vi "Authenticate user.vi"(8 "error in":errorcluster caption="에러 입력(에러 없음)", 9 "Password":string, 10 "User ID":string) -> (0 "error out":errorcluster caption="에러 출력", 1 "Verified?":bool)   [LabVIEW 2020]
uses:
  <vilib>/Utility/error.llb/DialogType.ctl
  <vilib>/addons/database/Connection.llb/Conn Execute.vi
  <vilib>/addons/database/Recordset.llb/Rec Get Recordset Properties (R).vi
  Variables/Global_Cal Info.vi
  <vilib>/addons/database/Recordset.llb/Rec Fetch String Data (R).vi
  <vilib>/addons/database/Recordset.llb/Rec Destroy - Connection.vi
  <vilib>/addons/database/NI_Database_API.lvlib
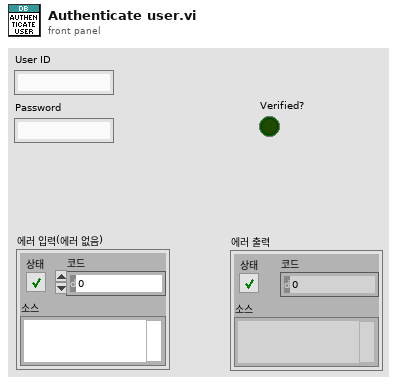
[diagram p1: front panel]
types:
  T1 = typedef "DialogType.ctl" = u16
  T2 = typedef "NI_Database_API.lvlib/Conn ObjectReference.ctl" = refnum<k1>
  T3 = typedef "NI_Database_API.lvlib/Rec ObjectReference.ctl" = refnum<k1>
  T4 = typedef "NI_Database_API.lvlib/Rec Properties.ctl" = cluster{"column count":i32, "record index":i32, "record count":i32, "bof?":bool, "eof?":bool, "cursor type":T5, "cache size":i32, "state":enum16{"closed", "open"}}
  T5 = typedef "NI_Database_API.lvlib/DB Tools Cursor Type.ctl" = enum16{"forward-only", "keyset", "dynamic", "static"}
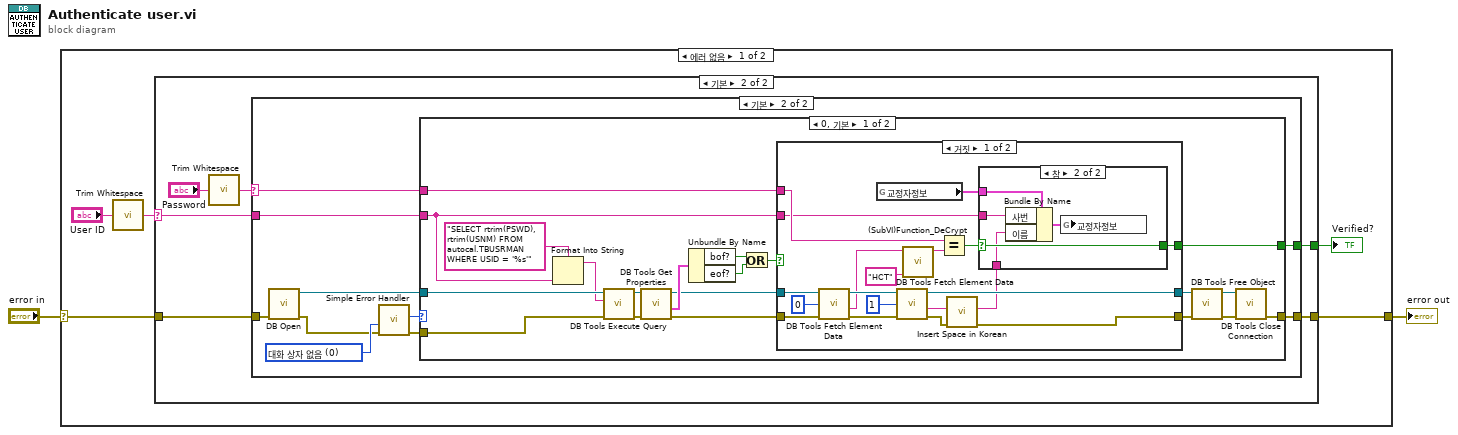
[diagram p0: block diagram]
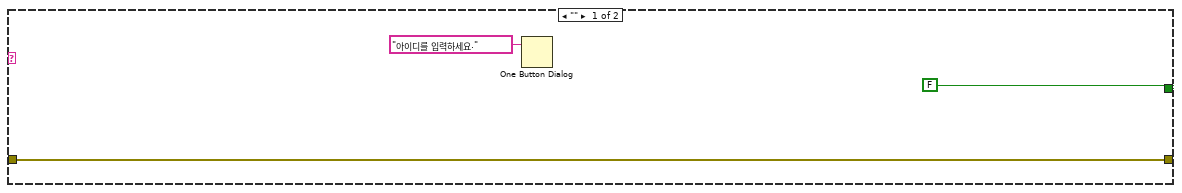
[diagram p2: hidden frame]
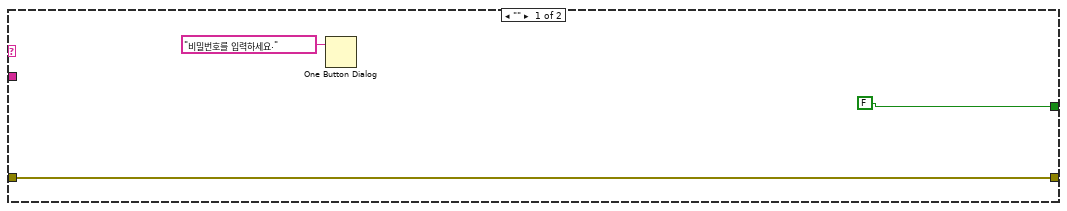
[diagram p3: hidden frame]
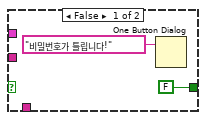
[diagram p4: hidden frame]
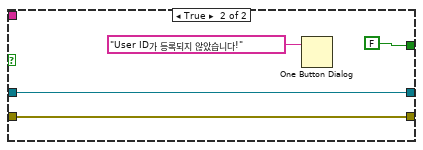
[diagram p5: hidden frame]
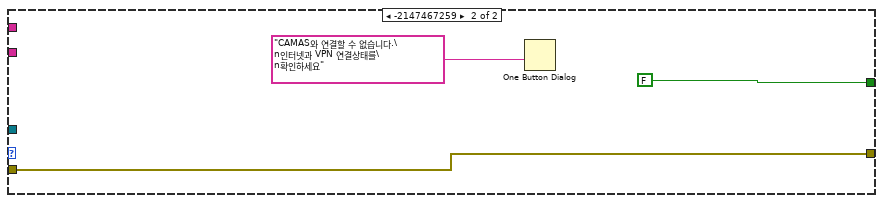
[diagram p6: hidden frame]
diagram:
  n1 = case shown="에러 없음" "error in" {
    selector: "error in" -> [w5 w83]
    tunnel: [w6 w83] -> w2
    frame No Error {
      n2 = call <vilib>:"Trim Whitespace.vi"("string"="User ID") -> ("trimmed string"=w3:string)  [unwired: 1 in]
      n3 = case shown="기본" w3 {
        selector: w3 -> [_ w13]
        tunnel: [w9 w16] -> w6
        tunnel: w5 -> [w9 w15]
        tunnel: [FALSE w14] -> w4
        frame "" {
          n4 = One Button Dialog(message="아이디를 입력하세요." ("메시지")) -> ()  [unwired: 1 in, 1 out]
        }
        frame Default {
          n5 = call <vilib>:"Trim Whitespace.vi"("string"="Password") -> ("trimmed string"=w11:string)  [unwired: 1 in]
          n6 = case shown="기본" w11 {
            selector: w11 -> [_ w20]
            tunnel: w13 -> [_ w27]
            tunnel: [w18 w29] -> w16
            tunnel: w15 -> [w18 w22]
            tunnel: [FALSE w28] -> w14
            frame "" {
              n7 = One Button Dialog(message="비밀번호를 입력하세요." ("메시지")) -> ()  [unwired: 1 in, 1 out]
            }
            frame Default {
              w25 = T1 0 items=["대화 상자 없음", "확인 메시지", "메시지 지속 또는 정지", "확인 메시지 + 경고", "지속/정지 + 경고"] ("type of dialog (OK msg:1)")
              n8 = call "DB Open.vi"("에러 입력"=w22) -> ("에러 출력"=w21:errorcluster, "참조 번호 출력"=w23:T2)  [unwired: 9 in]
              n9 = call <vilib>:"Simple Error Handler.vi"("type of dialog (OK msg:1)"=w25, "error in (no error)"=w21) -> ("code out"=w24:i32, "error out"=w26:errorcluster)  [unwired: 3 in, 3 out]
              n10 = case shown="0, 기본" w24 {
                tunnel: w20 -> [w41 _]
                tunnel: [w36 w82] -> w29
                tunnel: [w35 FALSE] -> w28
                tunnel: w27 -> [w31 _]
                tunnel: w26 -> [w34 w82]
                tunnel: w23 -> [w33 _]
                frame 0, Default {
                  n11 = Format Into String(format string="SELECT rtrim(PSWD), rtrim(USNM) FROM autocal.TBUSRMAN WHERE USID = '%s'" ("문자열"), w31) -> (resulting string=w30:string)  [unwired: 2 in, 1 out]
                  n12 = call-poly <vilib>:"DB Tools Execute Query.vi"("error in (no error)"=w34, "SQL query"=w30, "connection reference"=w33) -> ("error out"=w48:errorcluster, "recordset reference"=w49:T3)  [unwired: 5 in]
                  n13 = call-poly <vilib>:"DB Tools Get Properties.vi"("error in (no error)"=w48, "recordset reference"=w49) -> ("error out"=w43:errorcluster, "recordset properties"=w47:T4, "recordset reference out"=w42:T3)  [unwired: 3 in]
                  n14 = Unbundle By Name(w47) -> ("bof?"=w46:bool, "eof?"=w45:bool)
                  n15 = Or(x=w46, y=w45) -> (x .or. y?=w44:bool)
                  n16 = case shown="거짓" w44 {
                    tunnel: w43 -> [w68 w78]
                    tunnel: w42 -> [w64 w77]
                    tunnel: w41 -> [w62 _]
                    tunnel: [w53 w78] -> w40
                    tunnel: [w60 w77] -> w38
                    tunnel: [w59 FALSE] -> w35
                    tunnel: w31 -> [w58 _]
                    frame False {
                      n17 = call-poly <vilib>:"DB Tools Fetch Element Data.vi"("error in (no error)"=w68, "column index"=0, "recordset reference"=w64) -> ("error out"=w67:errorcluster, "data"=w57:string, "recordset reference out"=w63:T3)  [unwired: 4 in]
                      n18 = global read "Global_Cal Info.vi" "교정자정보"() -> (w50:cluster{"사번":string, "이름":string, "자격":string})
                      n19 = call-poly <vilib>:"DB Tools Fetch Element Data.vi"("error in (no error)"=w67, "column index"=1, "recordset reference"=w63) -> ("error out"=w54:errorcluster, "data"=w51:string, "recordset reference out"=w60:T3)  [unwired: 4 in]
                      n20 = call "(SubVI)Function_DeCrypt.vi"("Parameter"="HCT", "비밀번호"=w57) -> ("암호화된 비밀번호"=w56:string)  [unwired: 9 in]
                      n21 = Equal?(x=w62, y=w56) -> (x = y?=w61:bool)
                      n22 = call "Insert Space in Korean.vi"("error in (no error)"=w54, "in"=w51) -> ("error out"=w53:errorcluster, "out"=w52:string)  [unwired: 8 in]
                      n23 = case shown="참" w61 {
                        selector: w61 -> [_ w75]
                        tunnel: [FALSE w75] -> w59
                        tunnel: w52 -> [_ w74]
                        tunnel: w58 -> [_ w73]
                        tunnel: w50 -> [_ w71]
                        frame False {
                          n24 = One Button Dialog(message="비밀번호가 틀립니다!" ("메시지")) -> ()  [unwired: 1 in, 1 out]
                        }
                        frame True {
                          n25 = Bundle By Name(cluster=w71, "사번"=w73, "이름"=w74) -> (w72:cluster{"사번":string, "이름":string, "자격":string})
                          n26 = global write "Global_Cal Info.vi" "교정자정보"(w72) -> ()
                        }
                      }
                    }
                    frame True {
                      n27 = One Button Dialog(message="User ID가 등록되지 않았습니다!" ("메시지")) -> ()  [unwired: 1 in, 1 out]
                    }
                  }
                  n28 = call-poly <vilib>:"DB Tools Free Object.vi"("error in (no error)"=w40, "recordset reference"=w38) -> ("error out"=w39:errorcluster, "connection reference"=w37:T2)  [unwired: 8 in]
                  n29 = call <vilib>:"DB Tools Close Connection.vi"("error in (no error)"=w39, "connection reference"=w37) -> ("error out"=w36:errorcluster)  [unwired: 5 in]
                }
                frame -2147467259 {
                  n30 = One Button Dialog(message="CAMAS와 연결할 수 없습니다.\n인터넷과 VPN 연결상태를\n확인하세요" ("메시지")) -> ()  [unwired: 1 in, 1 out]
                }
              }
            }
          }
        }
      }
      "Verified?" <- w4
    }
    frame Error {
    }
  }
  "error out" <- w2
